vi "data need (SubVI).vi"(11 "요구":T1={"국번"="0", "커맨드"="01", "데이터 No."="00"}) -> (3 "출력":string)   [LabVIEW 2014]
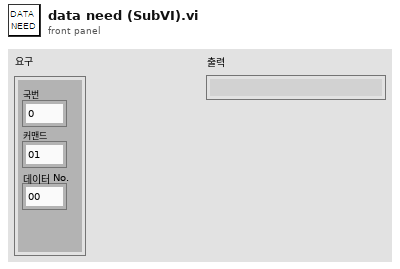
[diagram p1: front panel]
types:
  T1 = cluster{"국번":string, "커맨드":string, "데이터 No.":string}
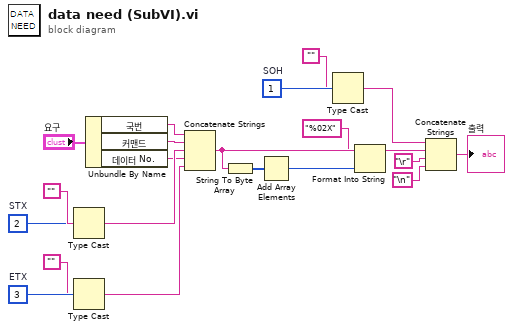
[diagram p0: block diagram]
diagram:
  w15 = u8 3  # ETX
  w11 = u8 2  # STX
  w6 = u8 1  # SOH
  n1 = Type Cast(type="", x=w11) -> (*(type *) &x=w13:string)
  n2 = Type Cast(type="", x=w15) -> (*(type *) &x=w16:string)
  n3 = Unbundle By Name("요구") -> ("국번"=w3:string, "커맨드"=w2:string, "데이터 No."=w1:string)
  n4 = Concatenate Strings(w3, w2, w13, w1, w16) -> (w10:string)
  n5 = String To Byte Array(string=w10) -> (unsigned byte array=w7:u8[])
  n6 = Add Array Elements(numeric array=w7) -> (sum=w8:u8)
  n7 = Type Cast(type="", x=w6) -> (*(type *) &x=w17:string)
  n8 = Format Into String(format string="%02X", initial string=w10, w8) -> (resulting string=w18:string)  [unwired: 1 in, 1 out]
  n9 = Concatenate Strings(w17, w18, "\r", "\n") -> (→"출력":string)
